vi "Day 17-Parse Example Possibilites.vi"() -> ()   [LabVIEW 2021]
uses:
  d2de5881-2a64-41ad-88cc-1dd0ed008079.vi
  <vilib>/Comparison/Less/Less Functor/Less Functor.lvclass
panel:
  out "sorted array":cluster{i32, i32}[](array[cluster])
  out "String":string
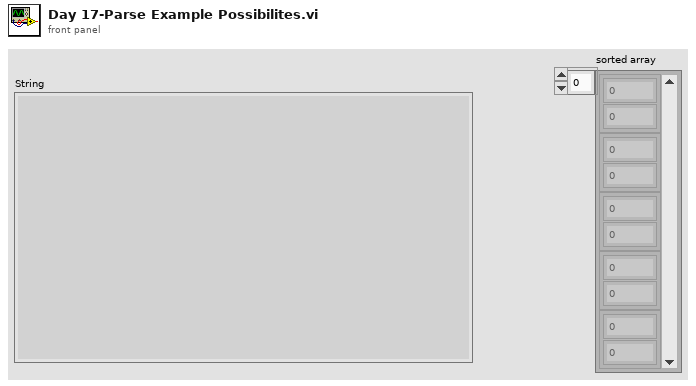
[diagram p1: front panel]
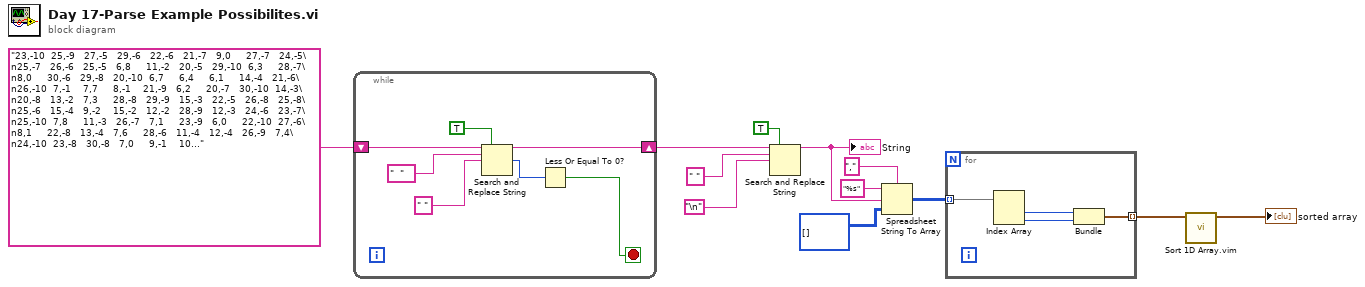
[diagram p0: block diagram]
diagram:
  n1 = while {
    shift-right: [w15] -> w11
    shift-left: "23,-10  25,-9   27,-5   29,-6   22,-6   21,-7   9,0     27,-7   24,-5\n25,-7   26,-6   25,-5   6,8     11,-2   20,-5   29,-10  6,3     28,-7\n8,0     30,-6   29,-8   20,-10  6,7     6,4     6,1     14,-4   21,-6\n26,-10  7,-1    7,7     8,-1    21,-9   6,2     20,-7   30,-10  14,-3\n20,-8   13,-2   7,3     28,-8   29,-9   15,-3   22,-5   26,-8   25,-8\n25,-6   15,-4   9,-2    15,-2   12,-2   28,-9   12,-3   24,-6   23,-7\n25,-10  7,8     11,-3   26,-7   7,1     23,-9   6,0     22,-10  27,-6\n8,1     22,-8   13,-4   7,6     28,-6   11,-4   12,-4   26,-9   7,4\n24,-10  23,-8   30,-8   7,0     9,-1    10,-1   26,-5   22,-9   6,5\n7,5     23,-6   28,-10  10,-2   11,-1   20,-9   14,-2   29,-7   13,-3\n23,-5   24,-8   27,-9   30,-7   28,-5   21,-10  7,9     6,6     21,-5\n27,-10  7,2     30,-9   21,-8   22,-7   24,-9   20,-6   6,9     29,-5\n8,-2    27,-8   30,-5   24,-7" -> [w19]
    stop <- w13 stop-if-true
    n2 = Search and Replace String(replace all?=TRUE ("replace all? (F)"), input string=w19, search string="  ", replace string=" " ("search string")) -> (result string=w15:string, number of replacements=w14:i32)  [unwired: 4 in, 2 out]
    n3 = Less Or Equal To 0?(x=w14) -> (x <= 0?=w13:bool)
  }
  n4 = Search and Replace String(replace all?=TRUE ("replace all? (F)"), input string=w11, search string=" ", replace string="\n") -> (result string=w7:string)  [unwired: 4 in, 3 out]
  "String" <- w7
  n5 = Spreadsheet String To Array(delimiter (Tab)=",", format string="%s", spreadsheet string=w7, array type (2D Dbl)=i32[][] []) -> (array=w3:i32[][])
  n6 = for {
    tunnel: w3 -> [w23] mode=indexing
    tunnel: [w20] -> w2 mode=indexing
    n7 = Index Array(array=w23) -> (element #1=w22:i32, element #2=w21:i32)  [unwired: 2 in]
    n8 = Bundle(w22, w21) -> (w20:cluster{i32, i32})  [unwired: 1 in]
  }
  n9 = call "Sort 1D Array.vim"("unsorted array"=w2) -> ("sorted array"=→"sorted array":cluster{i32, i32}[])  [unwired: 10 in]
